vi "读取测试数据.vi"(7 "停止":refnum<vi>, 8 "错误输入（无错误）":errorcluster, 11 "数据处理":refnum<queue>) -> (0 "错误输出":errorcluster, 3 "数据处理输出":refnum<queue>)   [LabVIEW 2020]
uses:
  viLib/QueueLib/QueueLib.lvlib
  VISA 2601B.vi
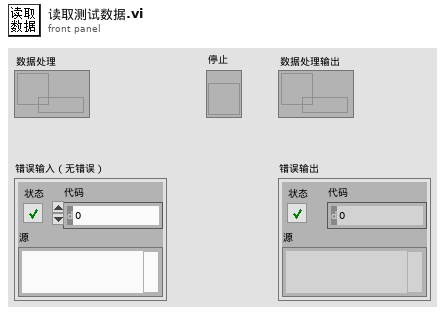
[diagram p1: front panel]
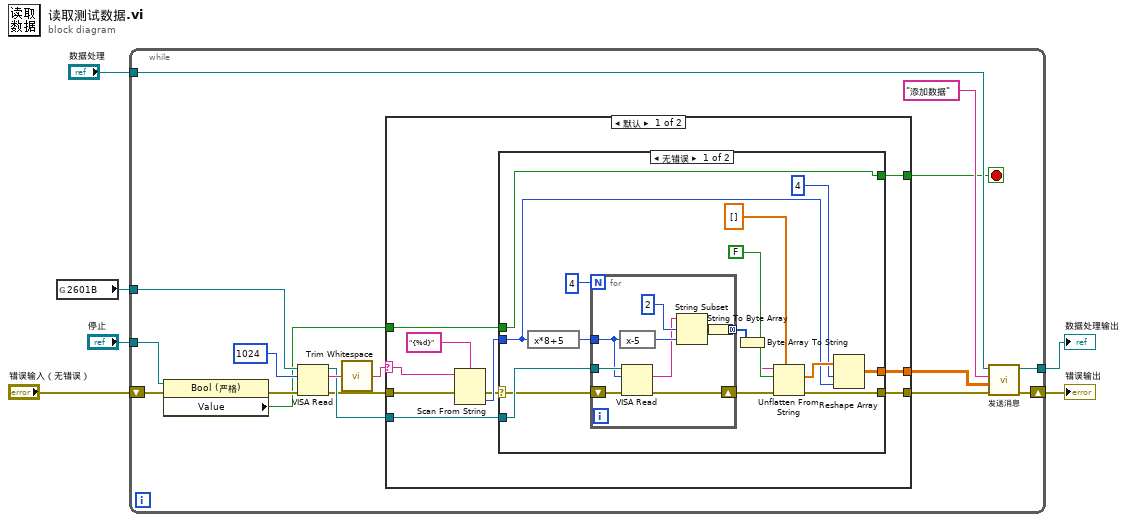
[diagram p0: block diagram]
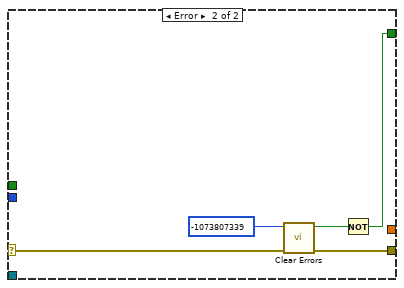
[diagram p2: hidden frame]
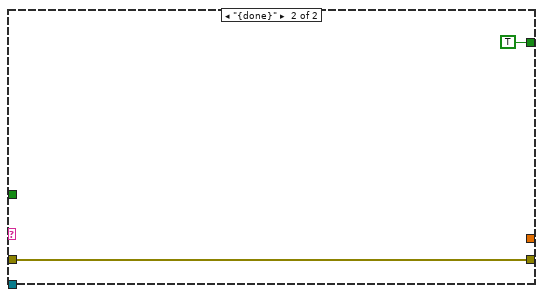
[diagram p3: hidden frame]
diagram:
  n1 = global read "VISA 2601B.vi" "2601B"() -> (w1:refnum<visa-resource-name>)
  n2 = while {
    tunnel: w1 -> [w18]
    tunnel: "数据处理" -> [w23]
    tunnel: [w22] -> w3
    shift-right: [w20] -> w5
    shift-left: "错误输入（无错误）" -> [w9]
    tunnel: "停止" -> [w11]
    stop <- w17 stop-if-true
    n3 = property class="Bool (严格)"(reference=w11, error in=w9) -> (error out=w8:errorcluster, "Value"=w7:bool)  [unwired: 1 out]
    n4 = VISA Read(VISA resource name=w18, byte count=u32 1024 ("字节总数"), error in (no error)=w8) -> (VISA resource name out=w14:refnum<visa-resource-name>, read buffer=w15:string, error out=w13:errorcluster)  [unwired: 1 out]
    n5 = call <vilib>:"Trim Whitespace.vi"("string"=w15) -> ("trimmed string"=w10:string)  [unwired: 1 in]
    n6 = case shown="默认" w10 {
      selector: w10 -> [w28 _]
      tunnel: w13 -> [w32 w64]
      tunnel: [w31 w64] -> w21
      tunnel: [w30 _] -> w16
      tunnel: w14 -> [w29 _]
      tunnel: [w25 TRUE] -> w17
      tunnel: w7 -> [w24 _]
      frame Default {
        n7 = Scan From String(format string="{%d}" ("格式字符串"), input string=w28, error in=w32) -> (error out=w26:errorcluster, output 1=w27:i32)  [unwired: 2 in, 2 out]
        n8 = case shown="无错误" w26 {
          selector: w26 -> [w40 w62]
          tunnel: w27 -> [w38 _]
          tunnel: [w44 w61] -> w31
          tunnel: [w42 _] -> w30
          tunnel: w29 -> [w48 _]
          tunnel: [w37 w58] -> w25
          tunnel: w24 -> [w37 _]
          frame No Error {
            n9 = expression code="x*8+5"(w38) -> (w41:i32)
            n10 = for {
              N: 4 -> [_]
              tunnel: w41 -> [w52]
              tunnel: [w49] -> w47 mode=concatenating
              shift-right: [w56] -> w45
              shift-left: w40 -> [w57]
              tunnel: w48 -> [w55]
              n11 = expression code="x-5"(w52) -> (w51:i32)
              n12 = VISA Read(VISA resource name=w55, byte count=w52, error in (no error)=w57) -> (read buffer=w50:string, error out=w56:errorcluster)  [unwired: 2 out]
              n13 = String Subset(string=w50, offset (0)=2 ("偏移量(0)"), length (rest)=w51) -> (substring=w53:string)
              n14 = String To Byte Array(string=w53) -> (unsigned byte array=w49:u8[])
            }
            n15 = Byte Array To String(unsigned byte array=w47) -> (string=w34:string)
            n16 = Unflatten From String(type=dbl[] [], binary string=w34, data includes array or string size? (T)=FALSE ("数据中包含数组或字符串大小？(T)"), error in (no error)=w45) -> (value=w43:dbl[], error out=w44:errorcluster)  [unwired: 1 in, 1 out]
            n17 = Reshape Array(w43, 4 ("维数大小"), w38) -> (w42:dbl[][])
          }
          frame Error {
            n18 = call <vilib>:"Clear Errors.vi"("error in (no error)"=w62, "specific error code to clear (0: all)"=-1073807339) -> ("error out"=w61:errorcluster, "specific error cleared?"=w59:bool)  [unwired: 4 in]
            n19 = Not(x=w59) -> (.not. x?=w58:bool)
          }
        }
      }
      frame "{done}" {
      }
    }
    n20 = call-poly "发送消息.vi"("错误输入（无错误）"=w21, "数据"=w16, "消息"="添加数据", "输入队列"=w23) -> ("错误输出"=w20:errorcluster, "输出队列"=w22:refnum<queue>)  [unwired: 6 in]
  }
  "错误输出" <- w5
  "数据处理输出" <- w3
